vi "Constants.vi"() -> ()   [LabVIEW 2018, in "CD_CI_Test Shared.lvlib"]
doc: "Use this Global VI to access the GUIDs assigned to the page resources of the Custom Device."
uses:
  CD_CI_Test Shared.lvlib
panel:
  in  "Tab Control":enum32{"GUIDS", "Constants", "Properties"}(tab)
  in  "CD_CI_Test":string="9a86ed75-7bef-49f2-b019-cd2b5c5ed659"
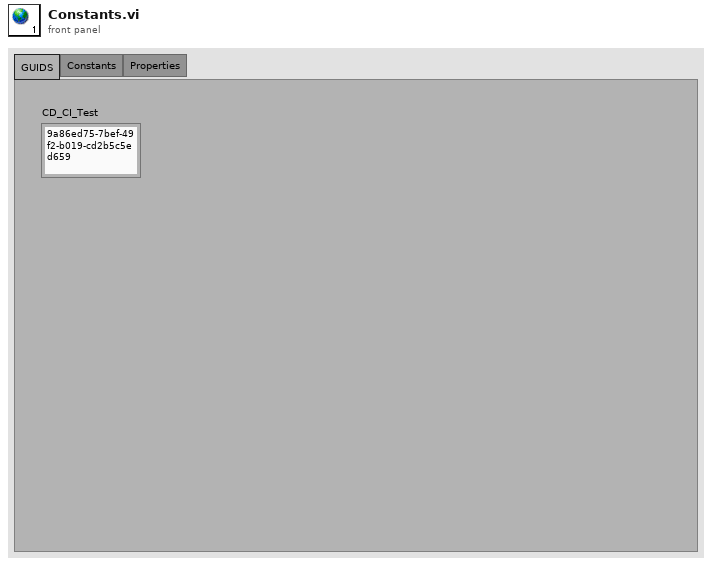
[diagram p1: front panel]
diagram:
